vi "Test_FormatValue_EmptyInput_NoErrorOut.vi"(8 "error in (no error)":errorcluster, 11 "TestCase in":refnum<class "TestVariantExtensions.lvclass">) -> (0 "error out":errorcluster, 3 "TestCase out":refnum<class "TestVariantExtensions.lvclass">)   [LabVIEW 2017, in "TestVariantExtensions.lvclass"]
uses:
  TestVariantExtensions.lvclass
  Source/Scalar Data to String.vi
  <vilib>/Utility/Data Type/Get Type Information.vi
  <vilib>/Utility/Data Type/Get Refnum Information.vi
  Source/VariantExtensions.lvlib
panel:
  out "Value as String":string
  out "Returned Error (None)":errorcluster
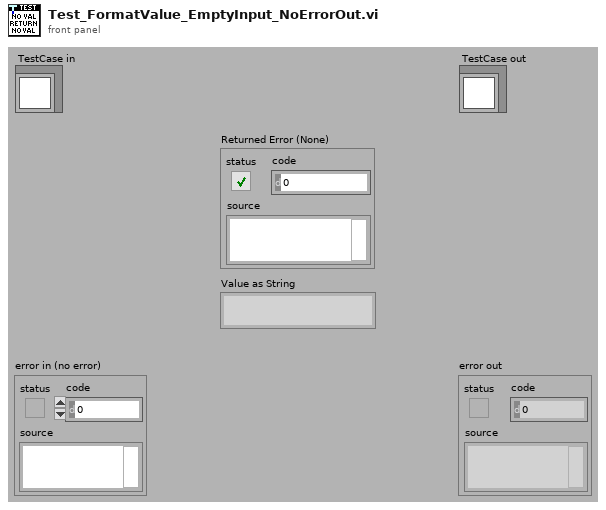
[diagram p1: front panel]
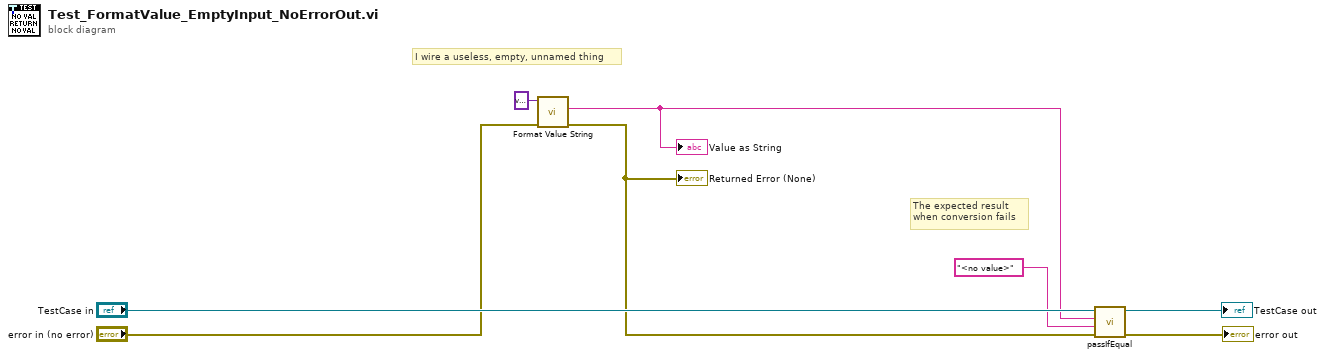
[diagram p0: block diagram]
diagram:
  # "The expected result\nwhen conversion fails"
  # "I wire a useless, empty, unnamed thing"
  n1 = call "Format Value String.vi"("error in (no error)"="error in (no error)", "Data"=variant) -> ("error out"=w2:errorcluster, "Value as String"=w5:string)  [unwired: 8 in]
  "Returned Error (None)" <- w2
  "Value as String" <- w5
  n2 = call-dynamic "passIfEqual.vi"("error in (no error)"=w2, "y"="<no value>", "x"=w5, "TestCase in"="TestCase in") -> ("error out"=→"error out":errorcluster, "TestCase out"=→"TestCase out":refnum<class "TestVariantExtensions.lvclass">)  [unwired: 6 in]
